vi "New ApplicationEventHandler.vi"(7 "Timeout Message Priority (Normal)":T1=enum."Normal", 8 "Timeout [ms]":i32=-1, 9 "Timeout Message":refnum<class "PreAddressedMsg.lvclass">, 10 "Registrations":T2[](array[typedef])) -> (0 "error out":errorcluster, 3 "ApplicationEventHandler":refnum<class "ApplicationEventHandler.lvclass">)   [LabVIEW 2015, in "ActorEvents.lvlib" / "ApplicationEventHandler.lvclass"]
uses:
  ApplicationEventHandler.lvclass
  AbstractMessages/PreAddressedMsg/PreAddressedMsg.lvclass
  <vilib>/event_ctls.llb/lveventtype.ctl
  <vilib>/ActorFramework/Message Enqueuer/Message Priority.ctl
  IEventHandler/IEventHandler.lvclass/IEventHandler.ctl
  ApplicationEventHandler.lvclass/ApplicationEventHandler.ctl
  <vilib>/Utility/error.llb/Error Cluster From Error Code.vi
  IEventHandler/IEventHandler.lvclass
  <vilib>/ActorFramework/Message Enqueuer/Message Enqueuer.lvclass
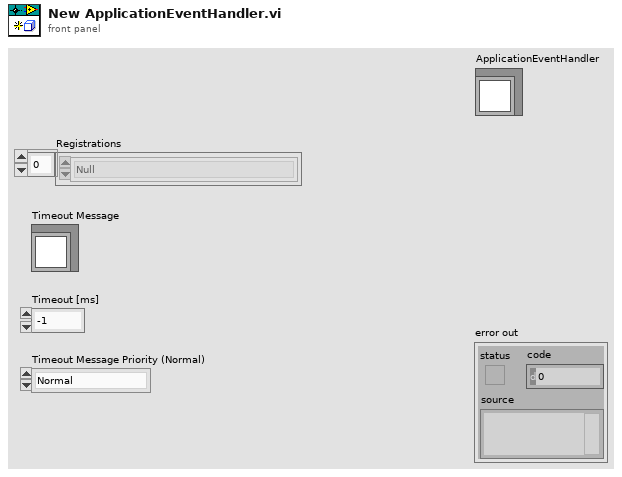
[diagram p1: front panel]
types:
  T1 = typedef "Actor Framework.lvlib/Message Enqueuer.lvclass/Message Priority.ctl" = enum16{"Low", "Normal", "High"}
  T2 = typedef "lveventtype.ctl" = enum32{"Null", "Timeout", "Annotation Menu Selection", "Annotation Menu Selection?", "App Instance Close", "App Instance Close?", "Autoscale Range Change", "Bookmark Info Change", "Cell Edit", "Cell Edit?", "Cursor Grab", "Cursor Grab?", "Cursor Menu Selection", "Cursor Menu Selection?", "Cursor Move", "Cursor Release", "Data Change", "Direction Change", "Display State Change", "Drag Ended", "Drag Enter", "Drag Leave", "Drag Over", "Drag Source Update", "Drag Starting", "Drag Starting?", "Drop", "Exec State Change", "Key Down", "Key Down?", "Key Repeat", "Key Repeat?", "Key Up", "Listbox Double Click", "Menu Activation?", "Menu Selection (App)", "Menu Selection? (App)", "Menu Selection (User)", "Mouse Down", "Mouse Down?", "Mouse Enter", "Mouse Leave", "Mouse Move", "Mouse Up", "Mouse Wheel", "NI Security User Change (App)", "Pane Size", "Panel Close", "Panel Close?", "Panel Resize", "Plot Attribute Change", "Scale Range Change", "Shortcut Menu Activation?", "Shortcut Menu Selection (App)", "Shortcut Menu Selection? (App)", "Shortcut Menu Selection (User)", "Tree Double Click", "Tree Drag", "Tree Drag?", "Tree Drop", "Tree Drop?", "Tree Item Close", "Tree Item Close?", "Tree Item Open", "Tree Item Open?", "User Event", "Value Change"}
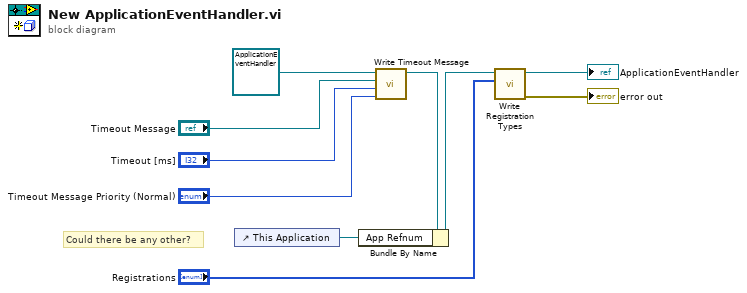
[diagram p0: block diagram]
diagram:
  # "Could there be any other?"
  n1 = control-ref of="This Application"() -> (w5:refnum<vi>)
  n2 = call "Write Timeout Message.vi"("Timeout Message Priority (Normal)"="Timeout Message Priority (Normal)", "Timeout [ms]"="Timeout [ms]", "Timeout Message"="Timeout Message", "IEventHandler in"=refnum<class "ApplicationEventHandler.lvclass"> refnum ("ApplicationEventHandler In")) -> ("IEventHandler out"=w9:refnum<class "ApplicationEventHandler.lvclass">)  [unwired: 7 in]
  n3 = Bundle By Name(cluster=w9, "App Refnum"=w5) -> (w10:refnum<class "ApplicationEventHandler.lvclass">)
  n4 = call "Write Registration Types.vi"("Requested Registration Types"="Registrations", "IEventHandler In"=w10) -> ("error out"=→"error out":errorcluster, "IEventHandler Out"=→"ApplicationEventHandler":refnum<class "ApplicationEventHandler.lvclass">)  [unwired: 8 in]
